vi "atMonochromator_logEvent_wavelength.vi"(8 "error in (no error)":errorcluster, 11 "logevent_wavelength_Ctl":T1) -> (0 "error out":errorcluster, 2 "function return":i32, 3 "logevent_wavelength_Ctl out":T1)   [LabVIEW 2016, in "SALLV_atMonochromator.lvlib"]
doc: "int atMonochromator_shm_logEvent_wavelengthLV(atMonochromator_logevent_wavelengthLV *logevent_wavelength_Ctl );"
uses:
  SALLV_atMonochromator.lvlib
  DataTypes/logevent_wavelength.ctl
  SALLV_atMonochromator.so
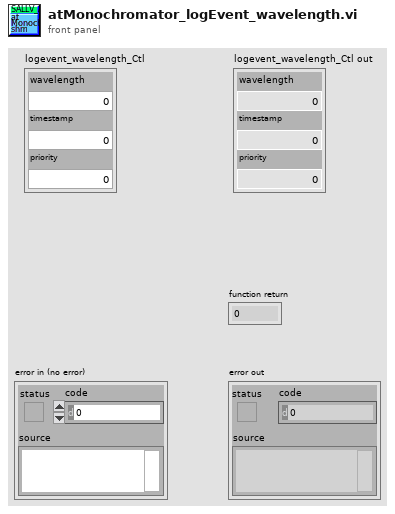
[diagram p1: front panel]
types:
  T1 = typedef "SALLV_atMonochromator.lvlib/logevent_wavelength.ctl" = cluster{"wavelength":sgl, "timestamp":dbl, "priority":i32}
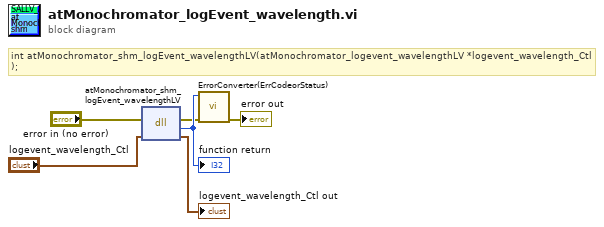
[diagram p0: block diagram]
diagram:
  # "int atMonochromator_shm_logEvent_wavelengthLV(atMonochromator_logevent_wavelengthLV *logevent_wavelength_Ctl );"
  n1 = dll-call lib="home/andres/Desktop/SAL_atMonochromator/SALLV_atMonochromator.*" fn="atMonochromator_shm_logEvent_wavelengthLV"(error in="error in (no error)", "logevent_wavelength_Ctl"="logevent_wavelength_Ctl") -> (error out=w2:errorcluster, w6:i32, "logevent_wavelength_Ctl"=→"logevent_wavelength_Ctl out":T1)  [unwired: 2 in, 1 out]
  "function return" <- w6
  n2 = call "ErrorConverter(ErrCodeorStatus).vi"("error in (no error)"=w2, "error code"=w6) -> ("error out"=→"error out":errorcluster)  [unwired: 9 in]
